vi "Do.vi"(8 "error in (no error)":errorcluster, 10 "Actor in":refnum<class "Actor.lvclass">, 11 "Configure FM Internal [FM] Msg":refnum<class "Configure FM Internal [FM] Msg.lvclass">) -> (0 "error out":errorcluster, 2 "Actor out":refnum<class "Actor.lvclass">)   [LabVIEW 2015, in "CS++Fgen.lvlib" / "Configure FM Internal [FM] Msg.lvclass"]
doc: "This VI delivers the message to the actor by calling the appropriate method(s) on the actor."
uses:
  Configure FM Internal [FM] Msg.lvclass
  <vilib>/ActorFramework/Actor/Actor.lvclass
  CS++Fgen/CS++Fgen.lvclass
  CSPP_Core/Actors/CS++PVMonitor Messages/CS++PVUpdate Msg/CS++PVUpdate Msg.lvclass/CS++PVUpdate Msg.ctl
  CSPP_Core/Classes/CS++ProcessVariables/ProcessVariable/PV.lvclass/PV.ctl
  Configure FM Internal [FM] Msg.lvclass/Configure FM Internal [FM] Msg.ctl
  CSPP_Core/Classes/CS++ProcessVariables/ProcessVariable/PV.lvclass
  CSPP_Core/Actors/CS++PVMonitor Messages/CS++PVUpdate Msg/CS++PVUpdate Msg.lvclass
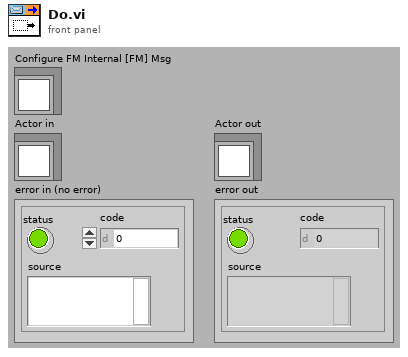
[diagram p1: front panel]
types:
  T1 = cluster{"peak deviation (100 Hz)":dbl[unit], "modulation frequency (1000 Hz)":dbl[unit], "modulation waveform (Sine)":i32}
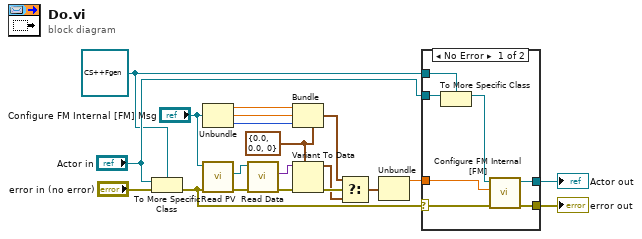
[diagram p0: block diagram]
diagram:
  w12 = T1 {"peak deviation (100 Hz)"=0.0, "modulation frequency (1000 Hz)"=0.0, "modulation waveform (Sine)"=0} ("Type")
  w16 = refnum<class "CS++Fgen.lvclass"> refnum ("Actor in")
  n1 = To More Specific Class(target class=w16, reference="Actor in", error in="error in (no error)") -> (error out=w5:errorcluster)  [unwired: 1 out]
  n2 = Unbundle ("Pre-Unbundler")("Configure FM Internal [FM] Msg") -> (w3:dbl[unit], w2:dbl[unit], w1:i32)
  n3 = call "Read PV.vi"("error in (no error)"=w5, "CS++PVUpdate Msg in"="Configure FM Internal [FM] Msg") -> ("error out"=w15:errorcluster, "PV"=w11:refnum<class "PV.lvclass">)  [unwired: 7 in, 1 out]
  n4 = call "Read Data.vi"("error in (no error)"=w15, "PV in"=w11) -> ("error out"=w9:errorcluster, "Data"=w10:variant)  [unwired: 7 in, 1 out]
  n5 = Bundle ("Pre-Bundler")(cluster=w12, "peak deviation (100 Hz)"=w3, "modulation frequency (1000 Hz)"=w2, "modulation waveform (Sine)"=w1) -> (w13:T1)
  n6 = Variant To Data(error in=w9, type=w12, Variant=w10) -> (data=w7:T1, error out=w14:errorcluster)
  n7 = Select ("MainSelect")(t=w13, s=w14, f=w7) -> (s? t:f=w8:T1)
  n8 = Unbundle ("Main-Unbundler")(w8) -> ("peak deviation (100 Hz)"=w4:dbl[unit])  [unwired: 2 out]
  n9 = case shown="No Error" w5 {
    selector: w5 -> [w25 w29]
    tunnel: [w27 w29] -> w19
    tunnel: [w26 w28] -> w18
    tunnel: "Actor in" -> [w24 w28]
    tunnel: w16 -> [w23 _]
    tunnel: w4 -> [w21 _]
    frame No Error {
      n10 = To More Specific Class(target class=w23, reference=w24) -> (specific class reference=w22:refnum<class "CS++Fgen.lvclass">)  [unwired: 1 in, 1 out]
      n11 = call "Configure FM Internal [FM].vi"("error in (no error)"=w25, "peak deviation (100 Hz)"=w21, "CS++Fgen in"=w22) -> ("error out"=w27:errorcluster, "CS++Fgen out"=w26:refnum<class "CS++Fgen.lvclass">)  [unwired: 7 in]
    }
    frame Error {
    }
  }
  "error out" <- w19
  "Actor out" <- w18
